vi "ServerNetworkInterfaceGlobalVariables.vi"() -> ()   [LabVIEW 2025]
panel:
  out "Network Interface Ready":bool
  out "Receive Data Queue":refnum<queue>
  out "Send Data Queue":refnum<queue>
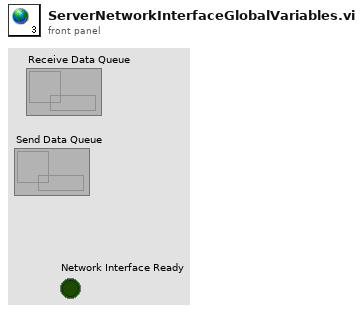
[diagram p1: front panel]
diagram:
